vi "ReadMultipleDataFromImage.vi"(8 "error in (no error)":errorcluster, 9 "Keys":string[](array[string]), 10 "Image In":T1, 11 "DataProcessor in":refnum<class "DataProcessor.lvclass">) -> (0 "error out":errorcluster, 1 "Values Out":string[](array[string]), 2 "Image Out":T1, 3 "DataProcessor out":refnum<class "DataProcessor.lvclass">)   [LabVIEW 2020, in "DataProcessor.lvlib" / "DataProcessor.lvclass"]
uses:
  DataProcessor.lvclass
  <vilib>/vision/Image Controls.llb/IMAQ Image.ctl
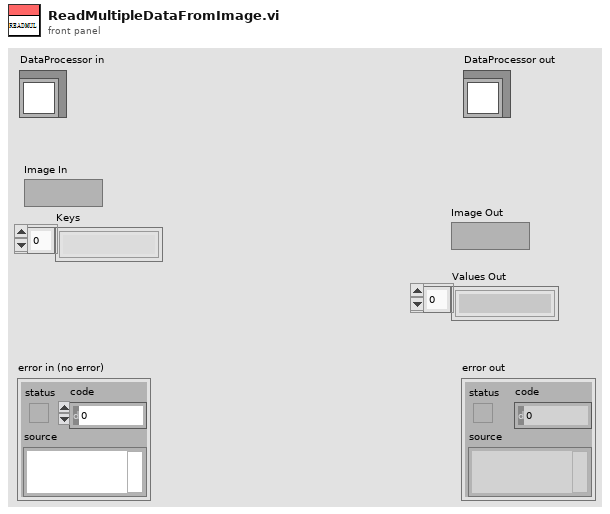
[diagram p1: front panel]
types:
  T1 = typedef "IMAQ Image.ctl" = refnum<image>
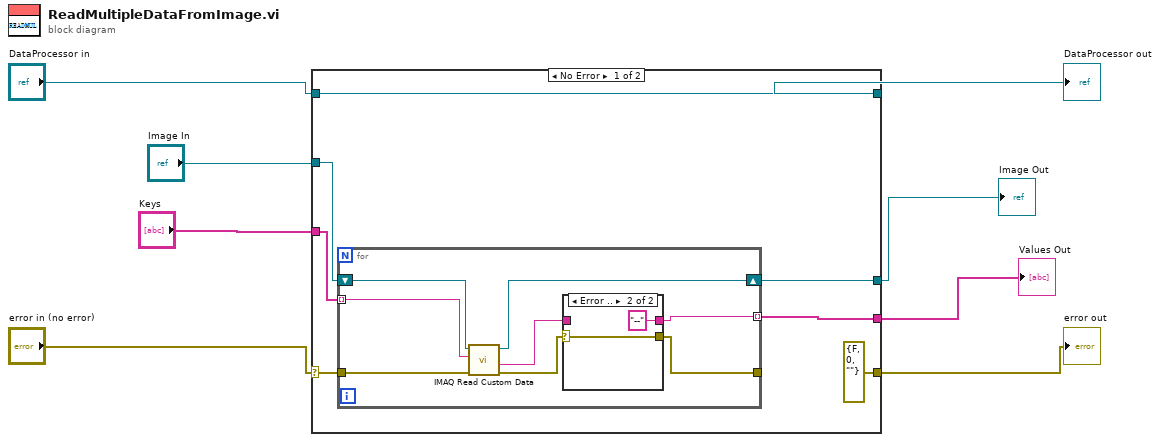
[diagram p0: block diagram]
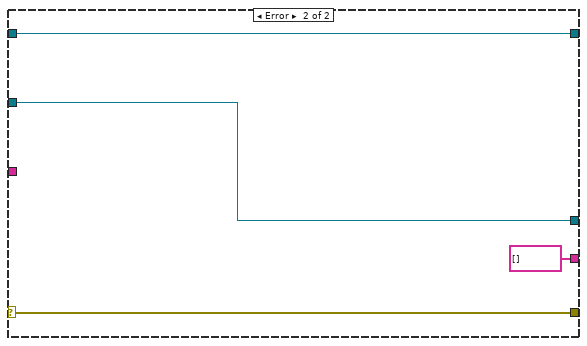
[diagram p3: hidden frame]
diagram:
  n1 = case shown="No Error" "error in (no error)" {
    selector: "error in (no error)" -> [w14 w31]
    tunnel: [errorcluster {"status"=FALSE, "code"=0, "source"=""} ("error IO") w31] -> w5
    tunnel: [w15 w30] -> w4
    tunnel: "DataProcessor in" -> [w15 w30]
    tunnel: "Image In" -> [w13 w29]
    tunnel: "Keys" -> [w11 _]
    tunnel: [w12 w29] -> w2
    tunnel: [w10 string[] []] -> w1
    frame No Error {
      n2 = for {
        tunnel: w11 -> [w20] mode=indexing
        shift-right: [w21] -> w12
        shift-left: w13 -> [w22]
        tunnel: [w16] -> w10 mode=indexing
        tunnel: w14 -> [w23]
        tunnel: [w18] -> _
        n3 = call "IMAQ Read Custom Data"("error in (no error)"=w23, "Key"=w20, "Image"=w22) -> ("error out"=w19:errorcluster, "Custom Data Out"=w17:string, "Image (duplicate)"=w21:T1)  [unwired: 6 in]
        n4 = case shown="Error .." w19 {
          selector: w19 -> [w25 w27]
          tunnel: [w25 w27] -> w18
          tunnel: [w24 "--" ("Custom Data Out")] -> w16
          tunnel: w17 -> [w24 _]
          frame No Error {
          }
          frame Error {
          }
        }
      }
    }
    frame Error {
    }
  }
  "error out" <- w5
  "DataProcessor out" <- w4
  "Image Out" <- w2
  "Values Out" <- w1
